vi "PH_IEEE1394Camera.evt CamAttr Write.vi"(0 "i ref in":refnum<vi>, 1 "Instance":string, 2 "Set Num":dbl, 3 "Set String":string, 4 "Set Bool":bool, 5 "error in (no error)":errorcluster, 7 "Attribute Name":string) -> (14 "i ref out":refnum<vi>, 19 "error out":errorcluster)   [LabVIEW 2014, in "PH_IEEE1394Camera.lvlib"]
doc: "This VI sends a simple call for writing a camera attribute."
uses:
  PH_IEEE1394Camera.lvlib
  CSCore/CSSystem/CoreLib/CoreLib.short 2 byte array.vi
  CSCore/CSSystem/CoreLib/CoreLib.string 2 byte array.vi
  CSCore/CSSystem/CoreLib/CoreLib.double 2 byte array.vi
  CSCore/CSSystem/CoreLib/CoreLib.lvlib
  CSCore/BaseProcess/BaseProcess.lvlib
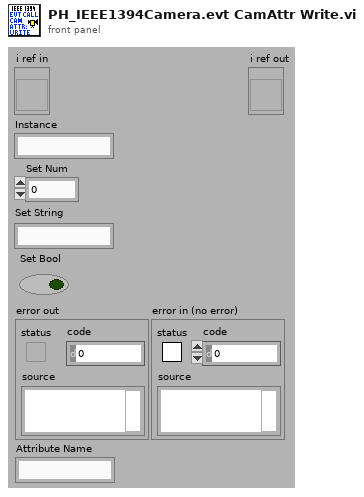
[diagram p1: front panel]
types:
  T1 = typedef "CoreDefs.rawDataType.ctl" = i8[]
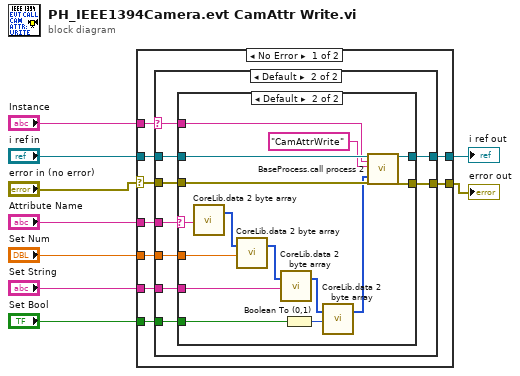
[diagram p0: block diagram]
diagram:
  n1 = case shown="No Error" "error in (no error)" {
    selector: "error in (no error)" -> [w14 w47]
    tunnel: [w18 w48] -> w5
    tunnel: [w17 w47] -> w4
    tunnel: "i ref in" -> [w16 w48]
    tunnel: "Instance" -> [w13 _]
    tunnel: "Set Bool" -> [w15 _]
    tunnel: "Set String" -> [w12 _]
    tunnel: "Set Num" -> [w11 _]
    tunnel: "Attribute Name" -> [w10 _]
    frame No Error {
      n2 = case shown="Default" w13 {
        selector: w13 -> [_ w22]
        tunnel: [w20 w29] -> w18
        tunnel: [w19 w28] -> w17
        tunnel: w16 -> [w20 w27]
        tunnel: w15 -> [_ w24]
        tunnel: w14 -> [w19 w26]
        tunnel: w12 -> [_ w25]
        tunnel: w11 -> [_ w23]
        tunnel: w10 -> [_ w21]
        frame "N/A" {
        }
        frame Default {
          n3 = case shown="Default" w21 {
            selector: w21 -> [_ w32]
            tunnel: [w31 w46] -> w29
            tunnel: [w30 w45] -> w28
            tunnel: w27 -> [w31 w44]
            tunnel: w26 -> [w30 w42]
            tunnel: w25 -> [_ w39]
            tunnel: w24 -> [_ w37]
            tunnel: w23 -> [_ w35]
            tunnel: w22 -> [_ w34]
            frame "", "N/A" {
            }
            frame Default {
              n4 = call-poly "CoreLib.data 2 byte array.vi"("string"=w32) -> ("byteArray out"=w33:T1)  [unwired: 18 in]
              n5 = call-poly "CoreLib.data 2 byte array.vi"("byteArray"=w33, "f64"=w35) -> ("byteArray out"=w36:T1)  [unwired: 17 in]
              n6 = call-poly "CoreLib.data 2 byte array.vi"("byteArray"=w36, "string"=w39) -> ("byteArray out"=w41:T1)  [unwired: 17 in]
              n7 = Boolean To (0,1)(Boolean=w37) -> (0, 1=w38:i16)
              n8 = call-poly "CoreLib.data 2 byte array.vi"("byteArray"=w41, "i16"=w38) -> ("byteArray out"=w40:T1)  [unwired: 17 in]
              n9 = call "BaseProcess.call process 2.vi"("i ref in"=w44, "Object"=w34, "Selector"="CamAttrWrite", "Data"=w40, "error in (no error)"=w42) -> ("i ref out"=w46:refnum<vi>, "error out"=w45:errorcluster)  [unwired: 13 in]
            }
          }
        }
      }
    }
    frame Error {
    }
  }
  "error out" <- w4
  "i ref out" <- w5
